vi "magnet locator panel.vi"() -> ()   [LabVIEW 2017]
uses:
  control panel globals.vi
panel:
  out "y":sgl format="%#.1f"
  out "x":sgl format="%#.1g"
  in  "autoscale":bool=TRUE
  out "rotation":dbl(knob)
  out "Tilt":dbl(knob) scale=0.0..180.0 scale format="%#.1f"
  out "Z":dbl(slide) scale=0.0..150.0 scale format="%#.1f"
  out "X,Y Position":cluster{dbl[], dbl[]}[](graph)
  in  "millisecond update":u32=100
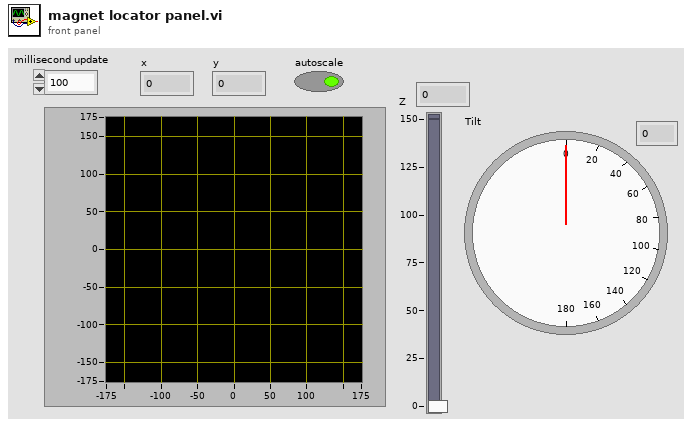
[diagram p1: front panel]
types:
  T1 = typedef "queue cluster.ctl" = cluster{"voltage":T2, "coil":T2, "mag":refnum<queue>, "accel":T2, "crossing":T2, "angle":T2, "pulse":T2, "mag0":T2, "fitLocation":T2}
  T2 = typedef "reading queue.ctl" = refnum<queue>
  T3 = typedef "reading.ctl" = cluster{"reading type":T4, "time":fxp<+,48,48>, "x":sgl, "y":sgl, "z":sgl, "XSUM":u8}
  T4 = typedef "readingType.ctl" = enum8{"SYNC", "DETVAL", "COILI", "MAGVEC", "ACCVEC", "CROSSING", "MAGVEC0", "MAGVEC1", "MAGVEC2", "MAGVEC3", "MAGVEC4", "MAGVEC5", "MAGVEC6", "MAGVEC7"}
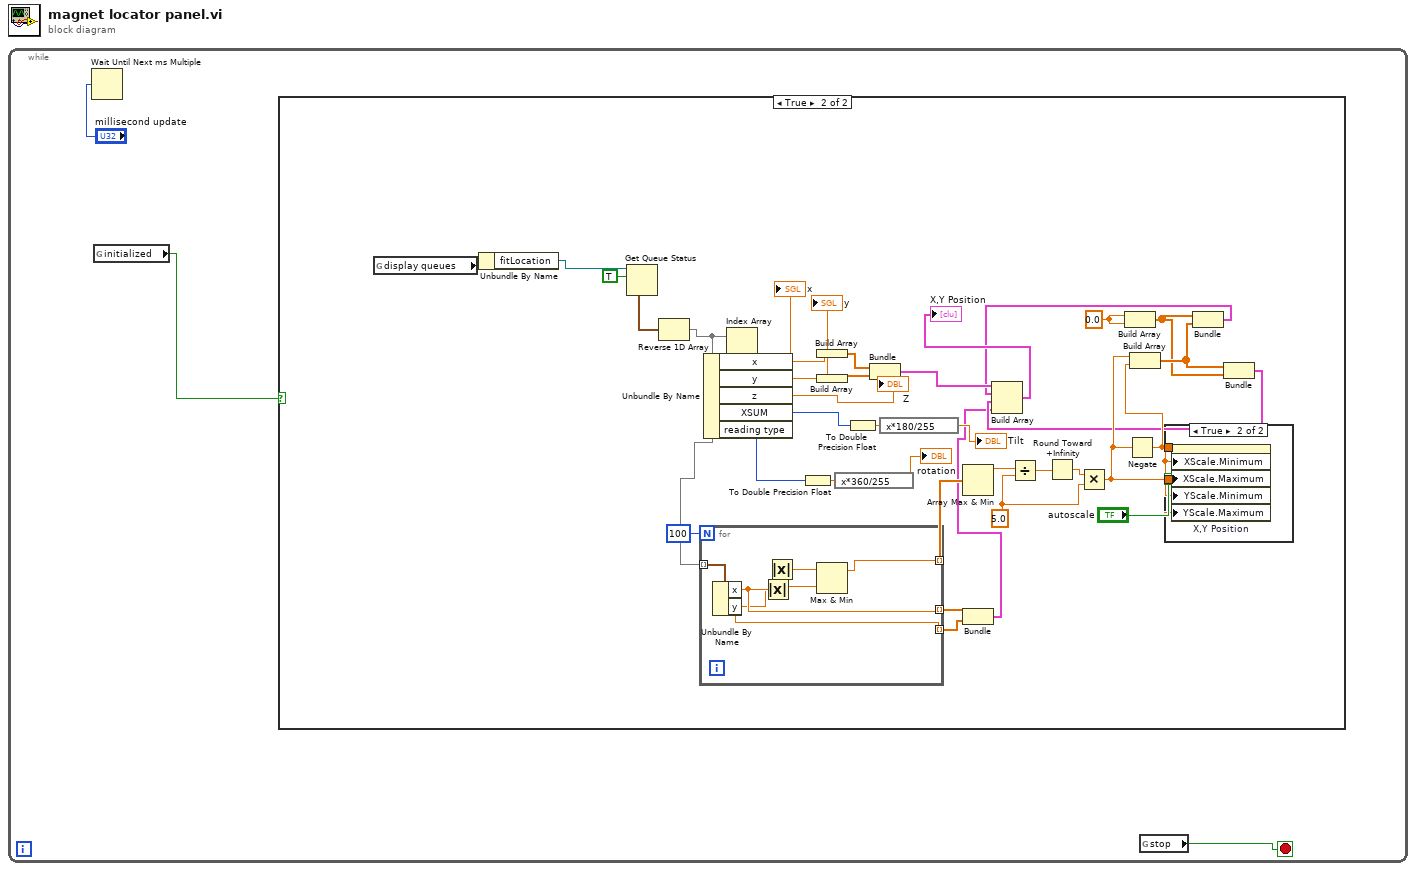
[diagram p0: block diagram]
diagram:
  n1 = while {
    stop <- w2 stop-if-true
    n2 = Wait Until Next ms Multiple(millisecond multiple="millisecond update") -> ()  [unwired: 1 out]
    n3 = global read "control panel globals.vi" "initialized"() -> (w1:bool)
    n4 = case shown="True" w1 {
      frame False {
      }
      frame True {
        w21 = 0.0
        w24 = sgl 5.0 ("y")
        n5 = global read "control panel globals.vi" "display queues"() -> (w39:T1)
        n6 = Unbundle By Name(w39) -> ("fitLocation"=w38:T2)
        n7 = Get Queue Status(queue=w38, return elements? (F)=TRUE) -> (elements=w36:T3[])  [unwired: 1 in, 7 out]
        n8 = Reverse 1D Array(array=w36) -> (reversed array=w29:T3[])
        n9 = for {
          N: 100 -> [_]
          tunnel: w29 -> [w47] mode=indexing
          tunnel: [w44] -> w28 mode=indexing
          tunnel: [w43] -> w7 mode=indexing
          tunnel: [w42] -> w6 mode=indexing
          n10 = Unbundle By Name(w47) -> ("x"=w43:sgl, "y"=w42:sgl)
          n11 = Absolute Value(x=w42) -> (abs(x)=w45:sgl)
          n12 = Absolute Value(x=w43) -> (abs(x)=w46:sgl)
          n13 = Max & Min(x=w46, y=w45) -> (max(x,y)=w44:sgl)  [unwired: 1 out]
        }
        n14 = Index Array(array=w29) -> (element=w35:T3)  [unwired: 1 in]
        n15 = Unbundle By Name(w35) -> ("x"=w34:sgl, "y"=w33:sgl, "z"=→"Z":sgl, "XSUM"=w14:u8, "reading type"=w10:T4)
        "x" <- w34
        "y" <- w33
        n16 = To Double Precision Float(number=w10) -> (double precision float=w11:dbl)
        n17 = Build Array(w34) -> (w32:sgl[])
        n18 = Build Array(w33) -> (w31:sgl[])
        n19 = expression code="x*360/255"(w11) -> (→"rotation":dbl)
        n20 = To Double Precision Float(number=w14) -> (double precision float=w13:dbl)
        n21 = Bundle(w32, w31) -> (w30:cluster{sgl[], sgl[]})  [unwired: 1 in]
        n22 = expression code="x*180/255"(w13) -> (→"Tilt":dbl)
        n23 = Array Max & Min(array=w28) -> (max value=w27:sgl)  [unwired: 3 out]
        n24 = Bundle(w7, w6) -> (w5:cluster{sgl[], sgl[]})  [unwired: 1 in]
        n25 = Divide(x=w27, y=w24) -> (x/y=w26:sgl)
        n26 = Round Toward +Infinity(x=w26) -> (ceil(x): smallest int >= x=w25:sgl)
        n27 = Multiply(x=w25, y=w24) -> (x*y=w23:sgl)
        n28 = Build Array(w21, w21) -> (w19:dbl[])
        n29 = Negate(x=w23) -> (-x=w22:sgl)
        n30 = Build Array(w23, w22) -> (w20:sgl[])
        n31 = case shown="True" "autoscale" {
          tunnel: w23 -> [_ w41]
          tunnel: w22 -> [_ w40]
          frame False {
          }
          frame True {
            n32 = property on="X,Y Position" class="XYGraph (strict)"("XScale.Minimum"=w40, "XScale.Maximum"=w41, "YScale.Minimum"=w40, "YScale.Maximum"=w41) -> ()  [unwired: 2 in, 2 out]
          }
        }
        n33 = Bundle(w19, w20) -> (w17:cluster{dbl[], sgl[]})  [unwired: 1 in]
        n34 = Bundle(w20, w19) -> (w16:cluster{sgl[], dbl[]})  [unwired: 1 in]
        n35 = Build Array(w30, w17, w16, w5) -> (→"X,Y Position":cluster{dbl[], dbl[]}[])
      }
    }
    n36 = global read "control panel globals.vi" "stop"() -> (w2:bool)
  }
